vi "PCO_RecorderDelete.vi"(8 "error in (no error)":errorcluster {"code" format="%x"}, 11 "phRec":u64) -> (0 "error out":errorcluster {"code" format="%x"}, 2 "ErrorMessage":i32 format="%x")   [LabVIEW 2019, in "Recorder.lvlib"]
doc: "<b>Description:</b>\nThis function deletes the recorder object. If necessary, it frees all allocated memory and resources. After this function has succeeded, it is possible to create a new recorder object.\nThe old recorder handle will be invalid.\nThe function will be rejected with an error if an acquisition is running.\n\n<b>Supported camera type:</b>\nAll cameras"
uses:
  Recorder.lvlib
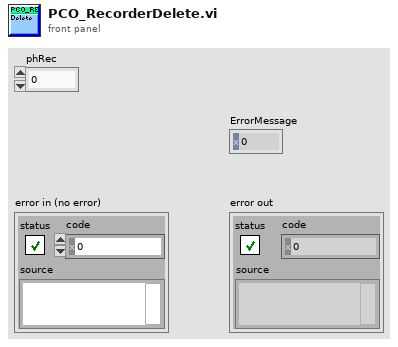
[diagram p1: front panel]
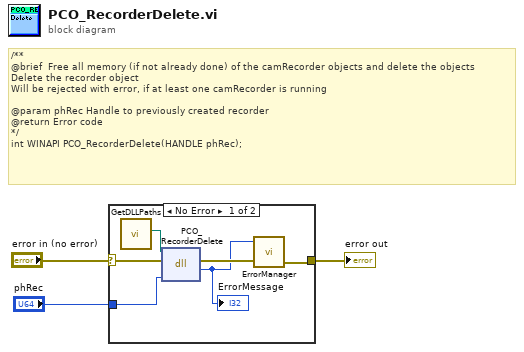
[diagram p0: block diagram]
diagram:
  # "/**\n@brief \tFree all memory (if not already done) of the camRecorder objects and delete the objects\nDelete the recorder object\nWill be rejected with error, if at least one camRecorder is running\n\n@param phRec Handle to previously created recorder\n@return Error code\n*/\nint WINAPI PCO_RecorderDelete(HANDLE phRec);"
  n1 = case shown="No Error" "error in (no error)" {
    selector: "error in (no error)" -> [w8 w10]
    tunnel: "phRec" -> [w9 _]
    tunnel: [w7 w10] -> w2
    frame No Error {
      n2 = call "GetDLLPaths.vi"() -> ("PCO_Recorder_Path"=w4:path)  [unwired: 9 in, 2 out]
      n3 = dll-call lib="?" fn="PCO_RecorderDelete"(path in=w4, error in=w8, "phRec"=w9) -> (error out=w6:errorcluster, "return type"=w5:i32)  [unwired: 2 in, 1 out]
      "ErrorMessage" <- w5
      n4 = call "ErrorManager.vi"("error in (no error)"=w6, "error code"=w5) -> ("error out"=w7:errorcluster)  [unwired: 3 in]
    }
    frame Error {
    }
  }
  "error out" <- w2
